vi "Actor Core.vi"(8 "error in":errorcluster, 11 "HIJ Vision Camera App Dialog in":refnum<class "HIJ Vision Camera App Dialog.lvclass">) -> (0 "error out":errorcluster, 3 "Actor out":refnum<class "Actor.lvclass">)   [LabVIEW 2020, in "HIJ Vision Camera App Dialog.lvlib" / "HIJ Vision Camera App Dialog.lvclass"]
doc: "(<B>Filename</B>: Actor Framework.lvlib:Actor.lvclass:Actor Core.vi)\n\nReceives messages to the actor, reacts to them, and initiates any error handling that may shut the actor down.\n\nDescendant classes may override this VI to append parallel tasks for the actor to complete while it handles messages. Overrides use the Call Parent Method node."
uses:
  HIJ Vision Camera App Dialog.lvclass
  C:/Users/AlexK/work/LabVIEW Programme/POLARIS CAM Log Abw und E/Submodules/Viewable Actor/ViewableActor/ViewableActor.lvclass
  C:/Program Files (x86)/National Instruments/LabVIEW 2020/vi.lib/ActorFramework/Actor/Actor.lvclass
  <vilib>/ActorFramework/Actor/Actor.lvclass
  HIJ Vision Camera App Dialog.lvclass/HIJ Vision Camera App Dialog.ctl
  <vilib>/ActorFramework/Actor/Actor.lvclass/Actor.ctl
  <vilib>/ActorFramework/Message Enqueuer/Message Enqueuer.lvclass/Message Enqueuer.ctl
  HIJ Vision Camera App Dialog Messages/Update Data befor stop Msg/Update Data befor stop Msg.lvclass/Update Data befor stop Msg.ctl
  HIJ Vision Application/HIJ Vision Application Messages/Write WorkDir Msg/Write WorkDir Msg.lvclass/Write WorkDir Msg.ctl
  HIJ Vision Camera App/HIJ Vision Camera App Messages/Write ConfigDir Msg/Write ConfigDir Msg.lvclass/Write ConfigDir Msg.ctl
  HIJ Vision Application/HIJ Vision Application Messages/Write Image Prefix Msg/Write Image Prefix Msg.lvclass/Write Image Prefix Msg.ctl
  HIJ Vision Camera App/HIJ Vision Camera App Messages/Start Aquisition Msg/Start Aquisition Msg.lvclass/Start Aquisition Msg.ctl
  Read ConfigDir.vi
  Read Prefix.vi
  Read WorkDir.vi
  Read Acquire.vi
  Read Camera Name.vi
  <vilib>/ActorFramework/Message Enqueuer/Init from Existing Queue.vi
  <vilib>/ActorFramework/Message Enqueuer/Enqueue.vi
  HIJ Vision Camera App Dialog Messages/Update Data befor stop Msg/Update Data befor stop Msg.lvclass
  C:/Program Files (x86)/National Instruments/LabVIEW 2020/vi.lib/ActorFramework/Message/Message.lvclass
  <vilib>/ActorFramework/Stop Msg/Stop Msg.lvclass
  HIJ Vision Application/HIJ Vision Application Messages/Write WorkDir Msg/Write WorkDir Msg.lvclass
  HIJ Vision Camera App/HIJ Vision Camera App Messages/Write ConfigDir Msg/Write ConfigDir Msg.lvclass
  HIJ Vision Application/HIJ Vision Application Messages/Write Image Prefix Msg/Write Image Prefix Msg.lvclass
  HIJ Vision Camera App/HIJ Vision Camera App Messages/Stop Aquisition Msg/Stop Aquisition Msg.lvclass
  HIJ Vision Camera App/HIJ Vision Camera App Messages/Start Aquisition Msg/Start Aquisition Msg.lvclass
  <vilib>/ActorFramework/Message Priority Queue/Priority Enqueue.vi
  <vilib>/ActorFramework/Message Enqueuer/Message Enqueuer.lvclass
  Viewable Actor/ViewableActor/ViewableActor.lvclass
  C:/Users/AlexK/work/LabVIEW Programme/POLARIS CAM Log Abw und E/Submodules/HIJ Vision/Application Base Actors/HIJ Vision Camera App Dialog/HIJ Vision Camera App Dialog/HIJ Vision Camera App Dialog.lvclass
panel:
  in  "stop":bool
  in  "Prefix":string
  in  "Acquire":bool
  in  "WorkDir":path=path "C:/Users/user/Desktop/test/WorkDir"
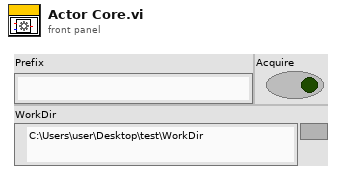
[diagram p1: front panel]
types:
  T1 = typedef "IMAQdx.ctl" = refnum<k21>
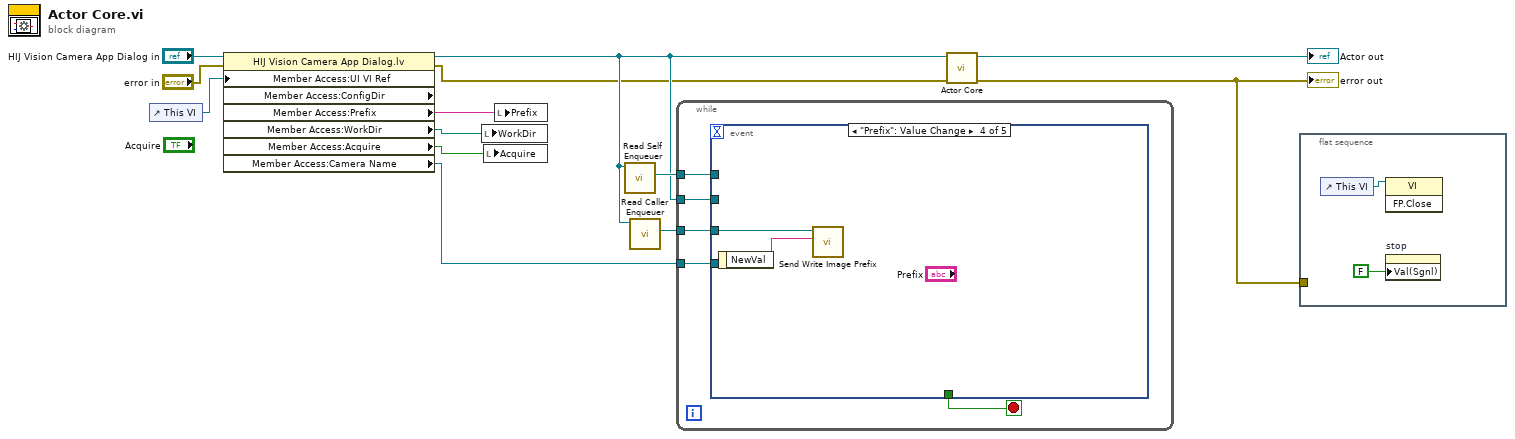
[diagram p0: block diagram]
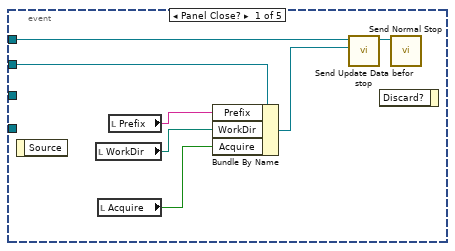
[diagram p2: hidden frame]
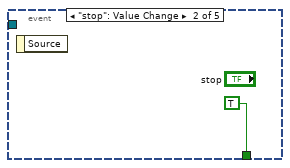
[diagram p3: hidden frame]
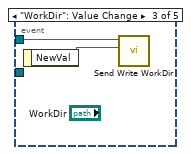
[diagram p4: hidden frame]
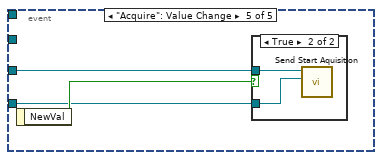
[diagram p5: hidden frame]
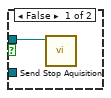
[diagram p6: hidden frame]
diagram:
  n1 = control-ref of="This VI"() -> (w9:refnum<vi>)
  n2 = property class="HIJ Vision Camera App Dialog.lv" props=["Member Access:UI VI Ref", "Member Access:ConfigDir", "Member Access:Prefix", "Member Access:WorkDir", "Member Access:Acquire", "Member Access:Camera Name"](reference="HIJ Vision Camera App Dialog in", error in="error in", "Member Access:UI VI Ref"=w9) -> (reference out=w3:refnum<class "HIJ Vision Camera App Dialog.lvclass">, error out=w2:errorcluster, "Member Access:Prefix"=w5:string, "Member Access:WorkDir"=w6:path, "Member Access:Acquire"=w4:bool, "Member Access:Camera Name"=w1:T1)  [unwired: 1 out]
  n3 = local write "WorkDir"(w6) -> ()
  n4 = local write "Acquire"(w4) -> ()
  n5 = local write "Prefix"(w5) -> ()
  n6 = call <vilib>:"Read Self Enqueuer.vi"("Actor"=w3) -> ("Self Enqueuer"=w12:refnum<class "Message Enqueuer.lvclass">)  [unwired: 10 in]
  n7 = call <vilib>:"Read Caller Enqueuer.vi"("Actor"=w3) -> ("Caller Enqueuer"=w7:refnum<class "Message Enqueuer.lvclass">)  [unwired: 10 in]
  n8 = while {
    tunnel: w12 -> [w18]
    tunnel: w7 -> [w16]
    tunnel: w3 -> [w15]
    tunnel: w1 -> [w14]
    stop <- w17 stop-if-true
    n9 = event shown="[3] \"Prefix\": Value Change" {
      selector: _ -> [_ _ _ _ _]
      dyn-events: _ -> [_ _ _ _ _]
      timeout: _ -> [_ _ _ _ _]
      tunnel: w18 -> [w21 _ _ _ _]
      tunnel: [_ TRUE _ _ _] -> w17
      tunnel: w16 -> [_ _ w28 w30 w32]
      tunnel: w15 -> [w25 _ _ _ _]
      tunnel: w14 -> [_ _ _ _ w31]
      event Panel Close? {
        n10 = event-data() -> ()  [unwired: 1 in, 1 out]
        n11 = local read "WorkDir"() -> (w23:path)
        n12 = local read "Acquire"() -> (w22:bool)
        n13 = local read "Prefix"() -> (w24:string)
        n14 = Bundle By Name(cluster=w25, "Prefix"=w24, "WorkDir"=w23, "Acquire"=w22) -> (w19:refnum<class "HIJ Vision Camera App Dialog.lvclass">)
        n15 = call "Send Update Data befor stop.vi"("Current State"=w19, "Message Enqueuer"=w21) -> ("Message Enqueuer out"=w20:refnum<class "Message Enqueuer.lvclass">)  [unwired: 8 in, 1 out]
        n16 = event-data() -> ()  [unwired: 2 in, 1 out]
        n17 = call <vilib>:"Send Normal Stop.vi"("Message Enqueuer"=w20) -> ()  [unwired: 10 in, 1 out]
      }
      event "stop": Value Change {
        n18 = event-data() -> ()  [unwired: 1 in, 1 out]
      }
      event "WorkDir": Value Change {
        n19 = event-data() -> ("NewVal"=w27:path)  [unwired: 1 in]
        n20 = call "Send Write WorkDir.vi"("Work Dir"=w27, "Message Enqueuer"=w28) -> ()  [unwired: 8 in, 2 out]
      }
      event "Prefix": Value Change {
        n21 = event-data() -> ("NewVal"=w29:string)  [unwired: 1 in]
        n22 = call "Send Write Image Prefix.vi"("Prefix"=w29, "Message Enqueuer"=w30) -> ()  [unwired: 8 in, 2 out]
      }
      event "Acquire": Value Change {
        n23 = event-data() -> ("NewVal"=w33:bool)  [unwired: 1 in]
        n24 = case shown="True" w33 {
          tunnel: w32 -> [w34 w36]
          tunnel: w31 -> [_ w35]
          frame False {
            n25 = call "Send Stop Aquisition.vi"("Message Enqueuer"=w34) -> ()  [unwired: 9 in, 2 out]
          }
          frame True {
            n26 = call "Send Start Aquisition.vi"("Camera"=w35, "Message Enqueuer"=w36) -> ()  [unwired: 8 in, 2 out]
          }
        }
      }
    }
  }
  n27 = call-parent "Actor Core.vi"("error in"=w2, "Actor in"=w3) -> ("error out"=w11:errorcluster, "Actor out"=→"Actor out":refnum<class "Actor.lvclass">)  [unwired: 8 in]
  "error out" <- w11
  n28 = flat-sequence {
    tunnel: w11 -> [_]
    frame #0 {
      n29 = control-ref of="This VI"() -> (w37:refnum<vi>)
      n30 = invoke class="VI" method="FP.Close"(reference=w37) -> ()  [unwired: 2 in, 3 out]
      n31 = property on="stop" class="Bool (strict)"("Val(Sgnl)"=FALSE ("Value (Signaling)")) -> ()  [unwired: 2 in, 2 out]
    }
  }
